vi "is_numeric_control.vi"(0 "Polished Command In":string, 5 "Cluster":cluster{"Start Offset":i32, "End offset":i32}, 11 "error in (no error)":errorcluster) -> (4 "Is Numeric":bool, 6 "Start Offset":i32, 8 "End offset":i32, 10 "Parameter Strings":string, 15 "error out":errorcluster)   [LabVIEW 2018]
uses:
  <vilib>/regexp/Match Regular Expression.xnode
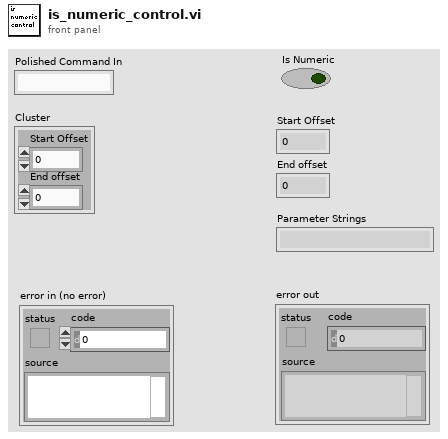
[diagram p1: front panel]
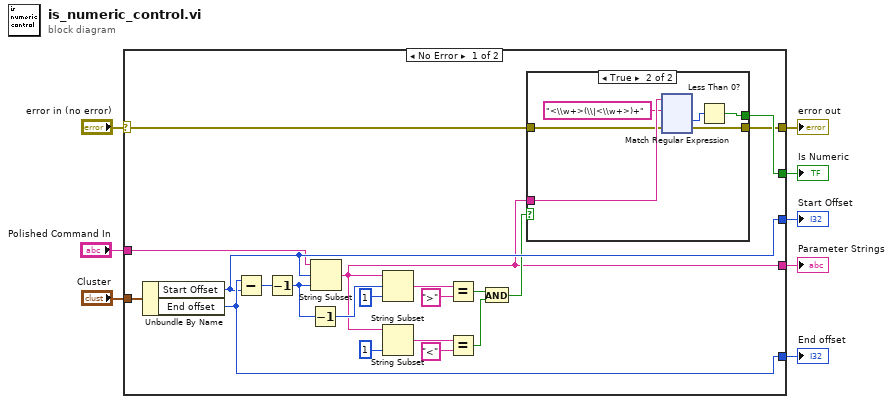
[diagram p0: block diagram]
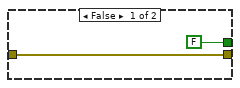
[diagram p2: hidden frame]
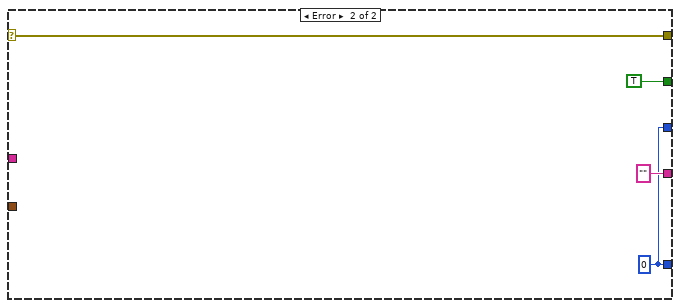
[diagram p3: hidden frame]
diagram:
  n1 = case shown="No Error" "error in (no error)" {
    selector: "error in (no error)" -> [w9 w151]
    tunnel: [w28 w148] -> w8
    tunnel: [w27 w148] -> w7
    tunnel: "Cluster" -> [w15 _]
    tunnel: "Polished Command In" -> [w14 _]
    tunnel: [w12 TRUE] -> w4
    tunnel: [w11 "" ("Polished Command In")] -> w3
    tunnel: [w10 w151] -> w1
    frame No Error {
      n2 = Unbundle By Name(w15) -> ("Start Offset"=w27:i32, "End offset"=w28:i32)
      n3 = Subtract(x=w28, y=w27) -> (x-y=w16:i32)
      n4 = Decrement(x=w16) -> (x-1=w19:i32)
      n5 = Decrement(x=w19) -> (x-1=w20:i32)
      n6 = String Subset(string=w14, offset (0)=w27, length (rest)=w19) -> (substring=w11:string)
      n7 = String Subset(string=w11, offset (0)=w20, length (rest)=1 ("length (rest)")) -> (substring=w21:string)
      n8 = String Subset(string=w11, length (rest)=1 ("length (rest)")) -> (substring=w23:string)  [unwired: 1 out]
      n9 = Equal?(x=w21, y=">") -> (x = y?=w25:bool)
      n10 = Equal?(x=w23, y="<") -> (x = y?=w26:bool)
      n11 = And(x=w25, y=w26) -> (x .and. y?=w13:bool)
      n12 = case shown="True" w13 {
        tunnel: [FALSE w33] -> w12
        tunnel: w11 -> [_ w36]
        tunnel: [w29 w32] -> w10
        tunnel: w9 -> [w29 w31]
        frame False {
        }
        frame True {
          n13 = xnode "Match Regular Expression"("input string"=w36, "regular expression"="<\\w+>(\\|<\\w+>)+", "error in"=w31) -> ("offset past match"=w34:i32, "error out"=w32:errorcluster)  [unwired: 1 in, 5 out]
          n14 = Less Than 0?(x=w34) -> (x < 0?=w33:bool)
        }
      }
    }
    frame Error {
      w148 = 0 ("Start Offset")
    }
  }
  "Parameter Strings" <- w3
  "End offset" <- w8
  "Start Offset" <- w7
  "Is Numeric" <- w4
  "error out" <- w1
